vi "USB2XXX_LINEX_MasterTest.vi"() -> ()   [LabVIEW 2010]
uses:
  PublicFiles/USB2XXX.dll
panel:
  in  "pInMsg 3":T1 {"Sync" format="%x"; "PID" format="%x"; "Data[0]" format="%x"; "Data[1]" format="%x"; "Data[2]" format="%x"; "Data[3]" format="%x"; "Data[4]" format="%x"; "Data[5]" format="%x"; "Data[6]" format="%x"; "Data[7]" format="%x"; "Check" format="%x"; "Reserve" format="%x"; "Reserve" format="%x"}
  in  "pInMsg 2":T1 {"Sync" format="%x"; "PID" format="%x"; "Data[0]" format="%x"; "Data[1]" format="%x"; "Data[2]" format="%x"; "Data[3]" format="%x"; "Data[4]" format="%x"; "Data[5]" format="%x"; "Data[6]" format="%x"; "Data[7]" format="%x"; "Check" format="%x"; "Reserve" format="%x"; "Reserve" format="%x"}
  out "pOutMsg":T2(array[cluster]) {"Sync" format="%x"; "PID" format="%x"; "Data[0]" format="%x"; "Data[1]" format="%x"; "Data[2]" format="%x"; "Data[3]" format="%x"; "Data[4]" format="%x"; "Data[5]" format="%x"; "Data[6]" format="%x"; "Data[7]" format="%x"; "Check" format="%x"}
  in  "pInMsg":T1 {"Sync" format="%x"; "PID" format="%x"; "Data[0]" format="%x"; "Data[1]" format="%x"; "Data[2]" format="%x"; "Data[3]" format="%x"; "Data[4]" format="%x"; "Data[5]" format="%x"; "Data[6]" format="%x"; "Data[7]" format="%x"; "Check" format="%x"; "Reserve" format="%x"; "Reserve" format="%x"}
  out "function return":i32
  in  "BaudRate":u32
  in  "Channel Index":u8(ring) items=["CH0"]
  in  "Device Index":i32(ring) items=["0", "1", "2", "3", "4", "5"]
  out "Flag(T:Write;F:Read)":bool=TRUE
  in  "stop":bool
  in  "Read":bool
  in  "Write":bool
  # "波特率一定要设置，否则程序可能出错"
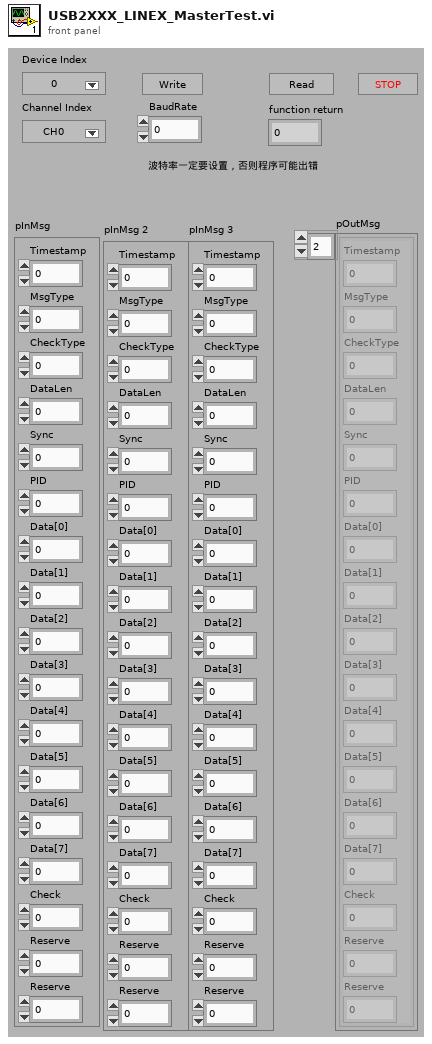
[diagram p1: front panel]
types:
  T1 = cluster{"Timestamp":u32, "MsgType":u8, "CheckType":u8, "DataLen":u8, "Sync":u8, "PID":u8, "Data[0]":u8, "Data[1]":u8, "Data[2]":u8, "Data[3]":u8, "Data[4]":u8, "Data[5]":u8, "Data[6]":u8, "Data[7]":u8, "Check":u8, "Reserve":u8, "Reserve":u8}
  T2 = cluster{"Timestamp":u32, "MsgType":u8, "CheckType":u8, "DataLen":u8, "Sync":u8, "PID":u8, "Data[0]":u8, "Data[1]":u8, "Data[2]":u8, "Data[3]":u8, "Data[4]":u8, "Data[5]":u8, "Data[6]":u8, "Data[7]":u8, "Check":u8, "Reserve":u8, "Reserve":u8}[]
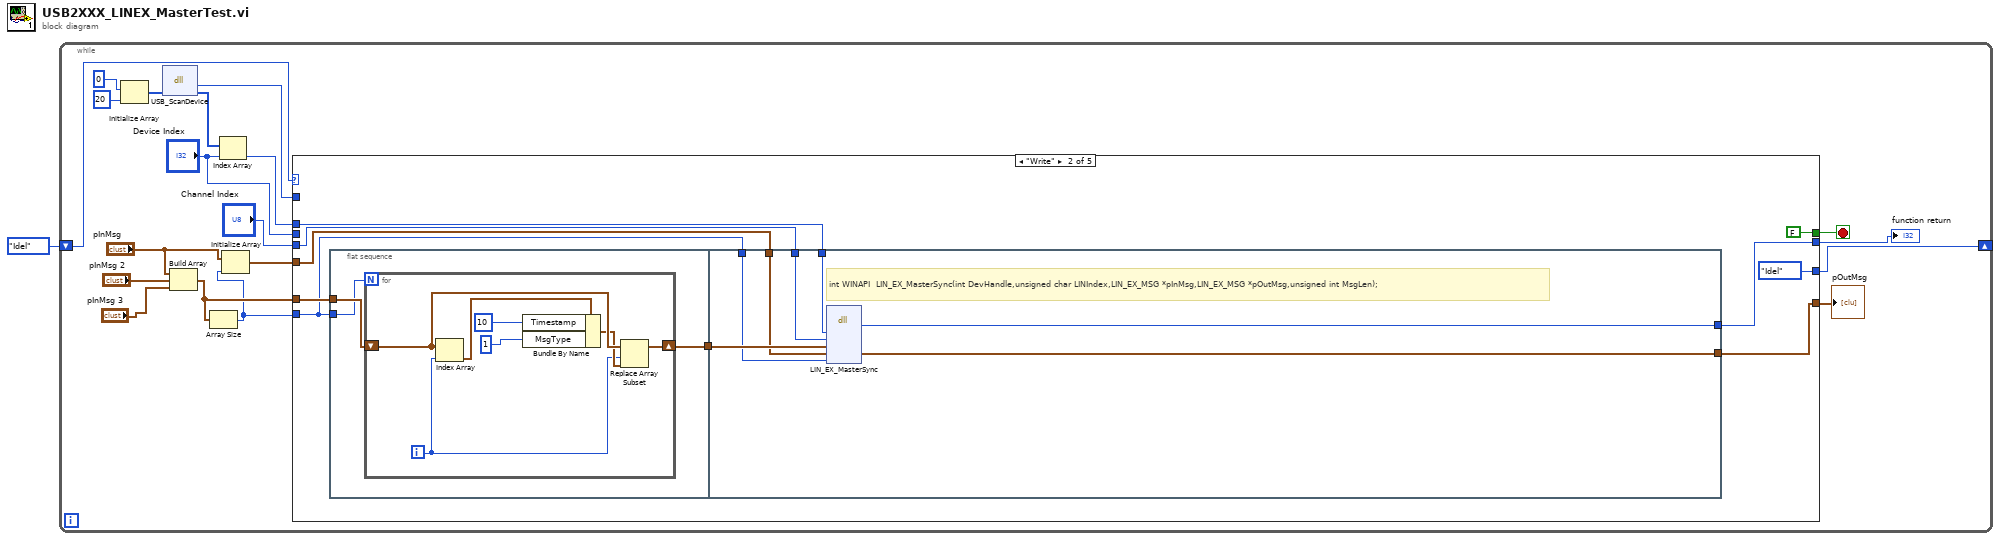
[diagram p0: block diagram]
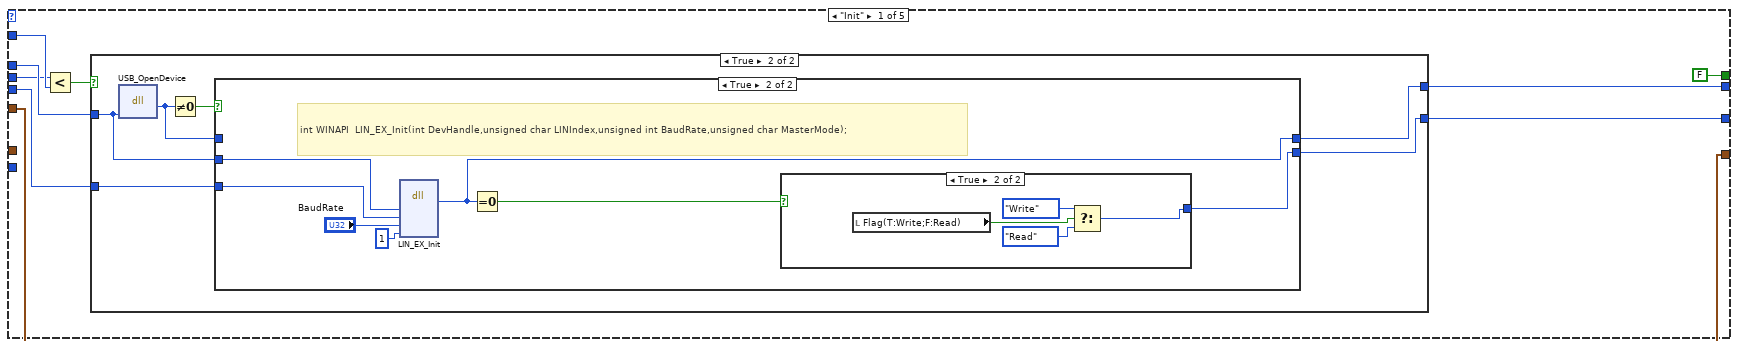
[diagram p2: hidden frame]
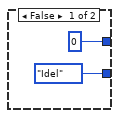
[diagram p3: hidden frame]
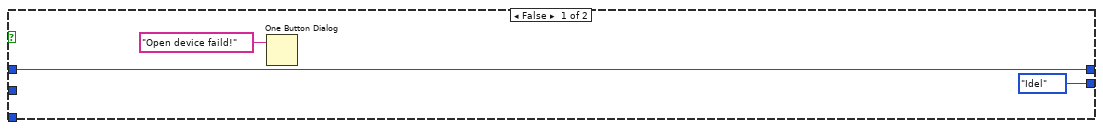
[diagram p4: hidden frame]
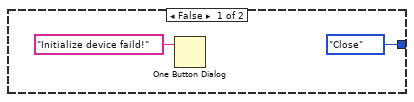
[diagram p5: hidden frame]
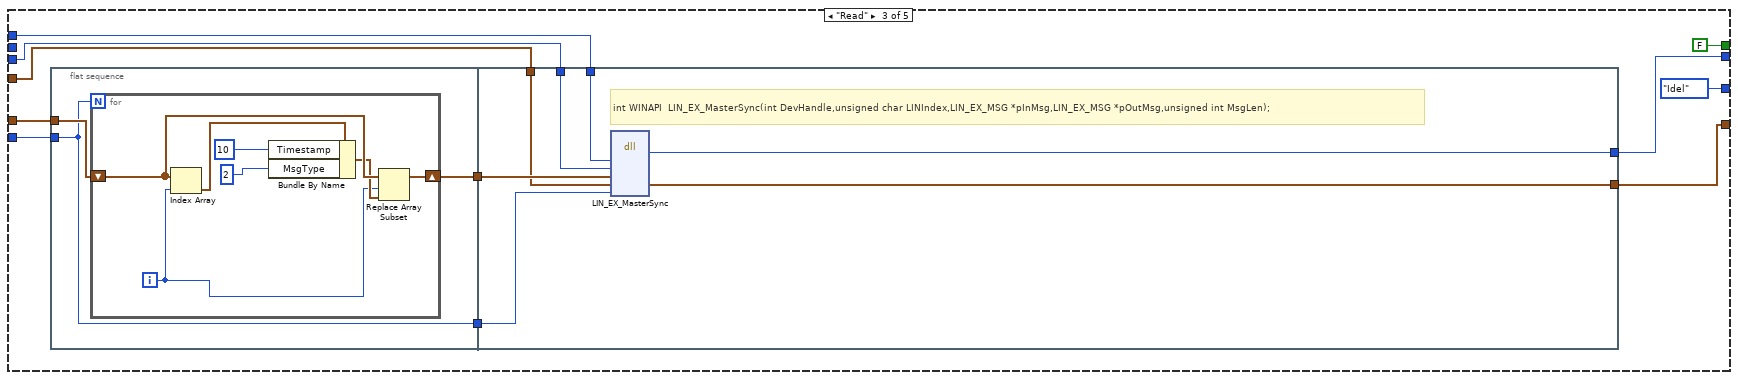
[diagram p6: hidden frame]
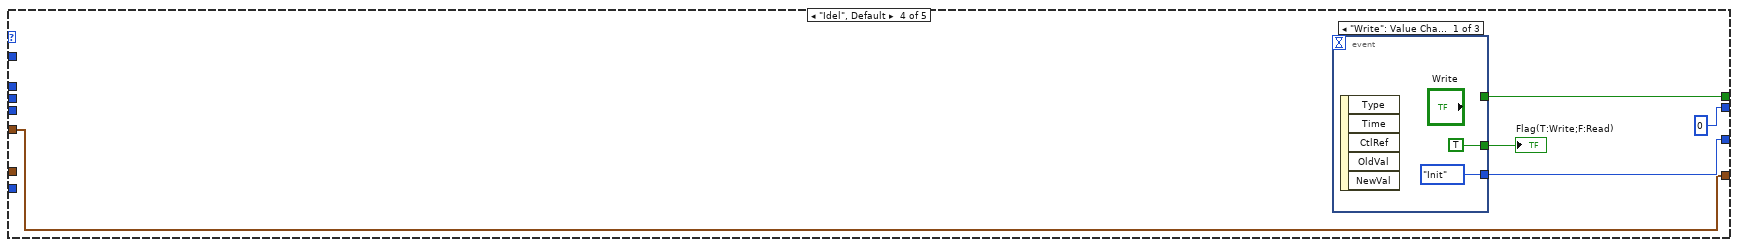
[diagram p7: hidden frame]
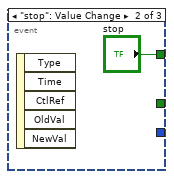
[diagram p8: hidden frame]
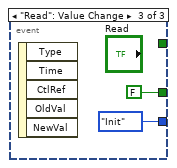
[diagram p9: hidden frame]
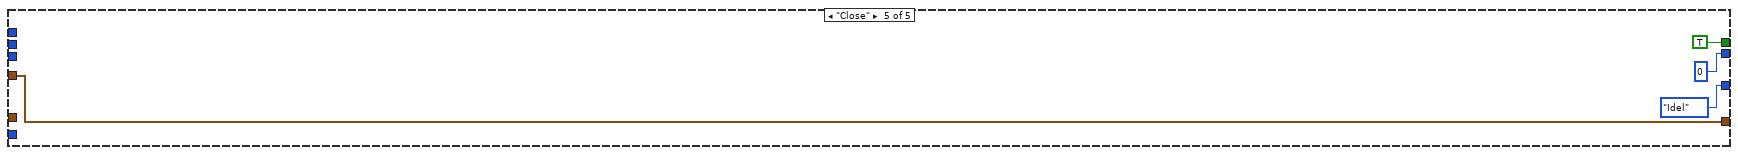
[diagram p10: hidden frame]
diagram:
  n1 = while {
    shift-right: [w19] -> _
    shift-left: enum16{"Init", "Write", "Read", "Idel", "Close"}."Idel" ("Enum") -> [w20]
    stop <- w17 stop-if-true
    n2 = Initialize Array(0, 20 ("dimension size")) -> (w16:i32[])
    n3 = dll-call lib="E:/OtherWork/STM32/USB2XXX_Example/trunk/Labview/PublicFiles/USB2XXX.dll" fn="USB_ScanDevice"("pDevNum"=w16) -> ("return type"=w12:i32, "pDevNum"=w13:i32[])  [unwired: 3 in, 2 out]
    n4 = Build Array("pInMsg", "pInMsg 2", "pInMsg 3") -> (w3:T2)
    n5 = Array Size(array=w3) -> (size(s)=w2:i32)
    n6 = Index Array(array=w13, index="Device Index") -> (element=w7:i32)
    n7 = Initialize Array("pInMsg", w2) -> (w10:T2)
    n8 = case shown="\"Write\"" w20 {
      tunnel: [w28 enum16{"Init", "Write", "Read", "Idel", "Close"}."Idel" ("Enum") enum16{"Init", "Write", "Read", "Idel", "Close"}."Idel" ("Enum") w111 enum16{"Init", "Write", "Read", "Idel", "Close"}."Idel" ("Enum")] -> w19
      tunnel: w7 -> [w24 w58 w87 _ _]
      tunnel: "Channel Index" -> [w27 w57 w86 _ _]
      tunnel: [FALSE FALSE FALSE w112 TRUE] -> w17
      tunnel: w12 -> [w25 _ _ _ _]
      tunnel: "Device Index" -> [w23 _ _ _ _]
      tunnel: w2 -> [_ w54 w84 _ _]
      tunnel: w10 -> [w22 w59 w85 w110 w120]
      tunnel: w3 -> [_ w61 w89 _ _]
      tunnel: [w22 w56 w81 w110 w120] -> w9
      tunnel: [w21 w55 w82 0 ("return type") 0 ("return type")] -> w8
      frame "Init" {
        n9 = Less?(x=w23, y=w25) -> (x < y?=w29:bool)
        n10 = case shown="True" w29 {
          tunnel: w24 -> [_ w35]
          tunnel: w27 -> [_ w36]
          tunnel: [enum16{"Init", "Write", "Read", "Idel", "Close"}."Idel" ("Enum") w34] -> w28
          tunnel: [0 ("return type") w33] -> w21
          frame False {
          }
          frame True {
            n11 = dll-call lib="E:/OtherWork/STM32/USB2XXX_Example/trunk/Labview/PublicFiles/USB2XXX.dll" fn="USB_OpenDevice"("DevIndex"=w35) -> ("return type"=w32:u8)  [unwired: 4 in, 2 out]
            n12 = Not Equal To 0?(x=w32) -> (x != 0?=w37:bool)
            n13 = case shown="True" w37 {
              tunnel: w36 -> [_ w43]
              tunnel: w35 -> [_ w44]
              tunnel: [enum16{"Init", "Write", "Read", "Idel", "Close"}."Idel" ("Enum") w46] -> w34
              tunnel: [w38 w41] -> w33
              tunnel: w32 -> [w38 _]
              frame False {
                n14 = One Button Dialog(message="Open device faild!") -> ()  [unwired: 1 in, 1 out]
              }
              frame True {
                # "int WINAPI  LIN_EX_Init(int DevHandle,unsigned char LINIndex,unsigned int BaudRate,unsigned char MasterMode);"
                n15 = dll-call lib="E:/OtherWork/STM32/USB2XXX_Example/trunk/Labview/PublicFiles/USB2XXX.dll" fn="LIN_EX_Init"("DevHandle"=w44, "LINIndex"=w43, "BaudRate"="BaudRate", "MasterMode"=u8 1) -> ("return type"=w41:i32)  [unwired: 7 in, 2 out]
                n16 = Equal To 0?(x=w41) -> (x = 0?=w47:bool)
                n17 = case shown="True" w47 {
                  tunnel: [enum16{"Init", "Write", "Read", "Idel", "Close"}."Close" ("Enum") w50] -> w46
                  frame False {
                    n18 = One Button Dialog(message="Initialize device faild!") -> ()  [unwired: 1 in, 1 out]
                  }
                  frame True {
                    n19 = local read "Flag(T:Write;F:Read)"() -> (w53:bool)
                    n20 = Select(t=enum16{"Init", "Write", "Read", "Idel", "Close"}."Write" ("Enum"), s=w53, f=enum16{"Init", "Write", "Read", "Idel", "Close"}."Read" ("Enum")) -> (s? t:f=w50:enum16{"Init", "Write", "Read", "Idel", "Close"})
                  }
                }
              }
            }
          }
        }
      }
      frame "Write" {
        n21 = flat-sequence {
          tunnel: w61 -> [w66]
          tunnel: w54 -> [w65]
          tunnel: [w64] -> w60
          tunnel: w60 -> [w80]
          tunnel: w59 -> [w79]
          tunnel: w58 -> [w78]
          tunnel: w57 -> [w77]
          tunnel: [w76] -> w56
          tunnel: [w75] -> w55
          tunnel: w54 -> [w74]
          frame #0 {
            n22 = for {
              N: w65 -> [_]
              shift-right: [w70] -> w64
              shift-left: w66 -> [w72]
              i -> [w69]
              n23 = Index Array(array=w72, index=w69) -> (element=w73:T1)
              n24 = Bundle By Name(cluster=w73, "Timestamp"=u32 10, "MsgType"=u8 1) -> (w71:T1)
              n25 = Replace Array Subset(array=w72, new element=w71, index=w69) -> (w70:T2)
            }
          }
          frame #1 {
            # "int WINAPI  LIN_EX_MasterSync(int DevHandle,unsigned char LINIndex,LIN_EX_MSG *pInMsg,LIN_EX_MSG *pOutMsg,unsigned int MsgLen);"
            n26 = dll-call lib="E:/OtherWork/STM32/USB2XXX_Example/trunk/Labview/PublicFiles/USB2XXX.dll" fn="LIN_EX_MasterSync"("DevHandle"=w78, "LINIndex"=w77, "pInMsg"=w80, "pOutMsg"=w79, "MsgLen"=w74) -> ("return type"=w75:i32, "pOutMsg"=w76:T2)  [unwired: 7 in, 2 out]
          }
        }
      }
      frame "Read" {
        n27 = flat-sequence {
          tunnel: w89 -> [w94]
          tunnel: [w93] -> w88
          tunnel: w84 -> [w92]
          tunnel: [w92] -> w83
          tunnel: w88 -> [w106]
          tunnel: w87 -> [w108]
          tunnel: w86 -> [w107]
          tunnel: w85 -> [w105]
          tunnel: w83 -> [w104]
          tunnel: [w103] -> w82
          tunnel: [w102] -> w81
          frame #0 {
            n28 = for {
              N: w92 -> [_]
              shift-right: [w98] -> w93
              shift-left: w94 -> [w100]
              i -> [w97]
              n29 = Index Array(array=w100, index=w97) -> (element=w101:T1)
              n30 = Bundle By Name(cluster=w101, "Timestamp"=u32 10, "MsgType"=u8 2) -> (w99:T1)
              n31 = Replace Array Subset(array=w100, new element=w99, index=w97) -> (w98:T2)
            }
          }
          frame #1 {
            # "int WINAPI  LIN_EX_MasterSync(int DevHandle,unsigned char LINIndex,LIN_EX_MSG *pInMsg,LIN_EX_MSG *pOutMsg,unsigned int MsgLen);"
            n32 = dll-call lib="E:/OtherWork/STM32/USB2XXX_Example/trunk/Labview/PublicFiles/USB2XXX.dll" fn="LIN_EX_MasterSync"("DevHandle"=w108, "LINIndex"=w107, "pInMsg"=w106, "pOutMsg"=w105, "MsgLen"=w104) -> ("return type"=w103:i32, "pOutMsg"=w102:T2)  [unwired: 7 in, 2 out]
          }
        }
      }
      frame "Idel", Default {
        n33 = event shown="[0] \"Write\": Value Change" {
          selector: _ -> [_ _ _]
          dyn-events: _ -> [_ _ _]
          timeout: _ -> [_ _ _]
          tunnel: [TRUE _ FALSE] -> w113
          tunnel: [_ "stop" _] -> w112
          tunnel: [enum16{"Init", "Write", "Read", "Idel", "Close"}."Init" ("Enum") _ enum16{"Init", "Write", "Read", "Idel", "Close"}."Init" ("Enum")] -> w111
          event "Write": Value Change {
            n34 = event-data() -> ()  [unwired: 1 in, 5 out]
          }
          event "stop": Value Change {
            n35 = event-data() -> ()  [unwired: 1 in, 5 out]
          }
          event "Read": Value Change {
            n36 = event-data() -> ()  [unwired: 1 in, 5 out]
          }
        }
        "Flag(T:Write;F:Read)" <- w113
      }
      frame "Close" {
      }
    }
    "pOutMsg" <- w9
    "function return" <- w8
  }
